vi "pickSurroundingPlatforms.vi"(9 "previousChoices":i32[][](array[numeric]), 10 "Goal \nplatform":i32, 11 "Start platform":i32) -> (3 "platform choices":i32[](array[numeric]))   [LabVIEW 2017]
panel:
  out "distance of \nchoices":dbl[](array[numeric])
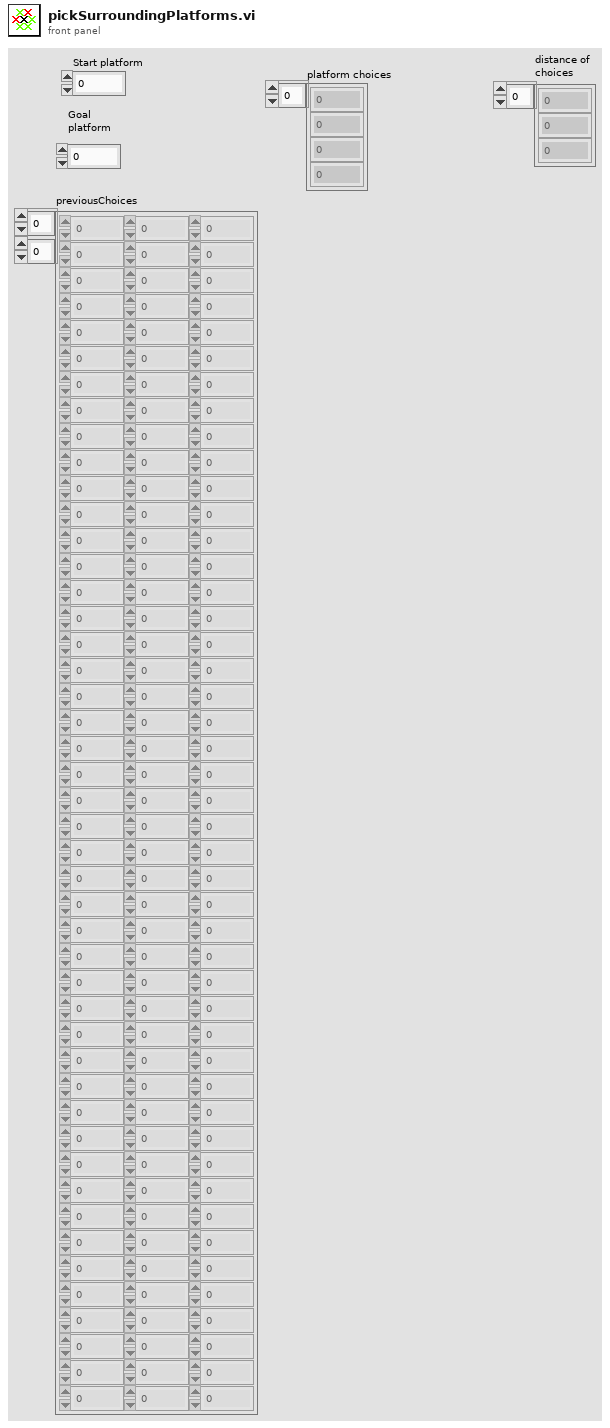
[diagram p1: front panel]
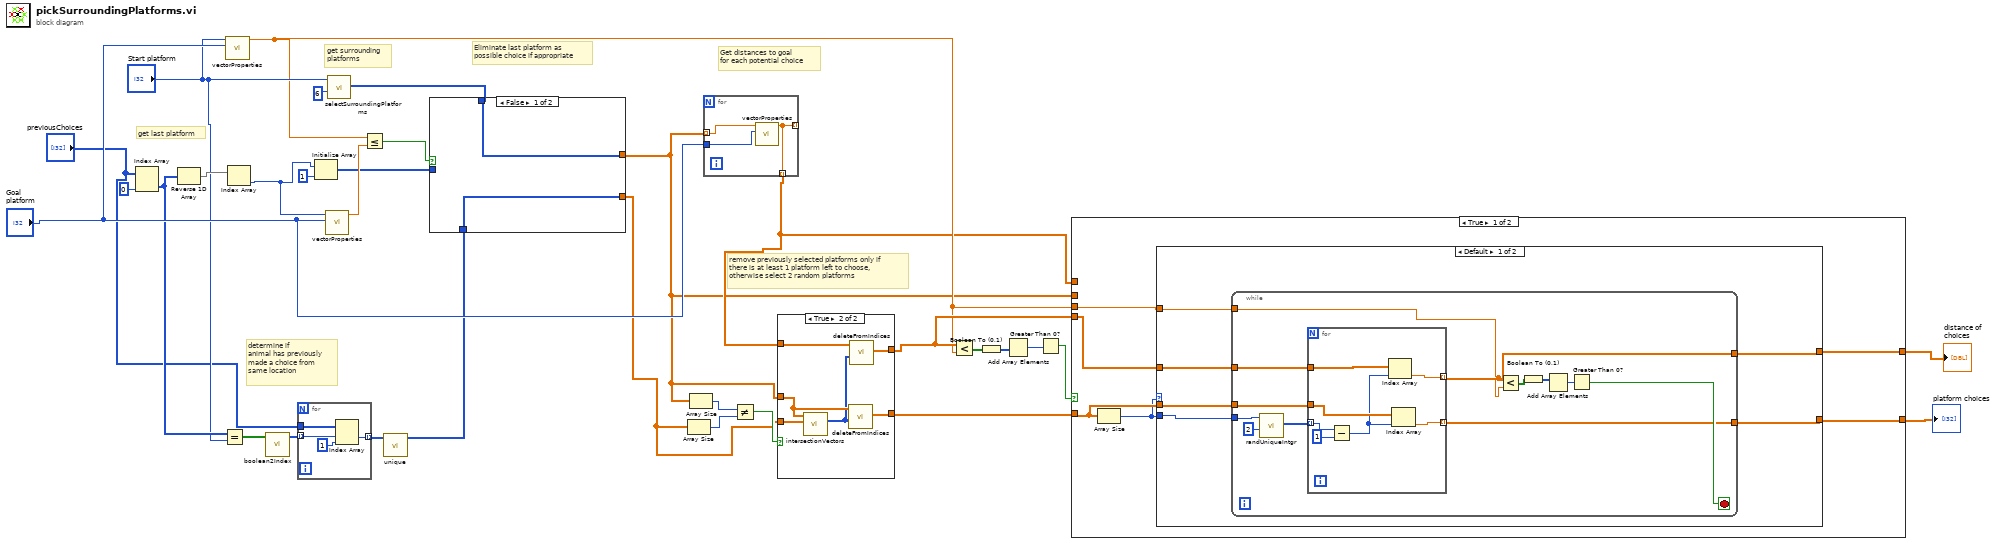
[diagram p0: block diagram]
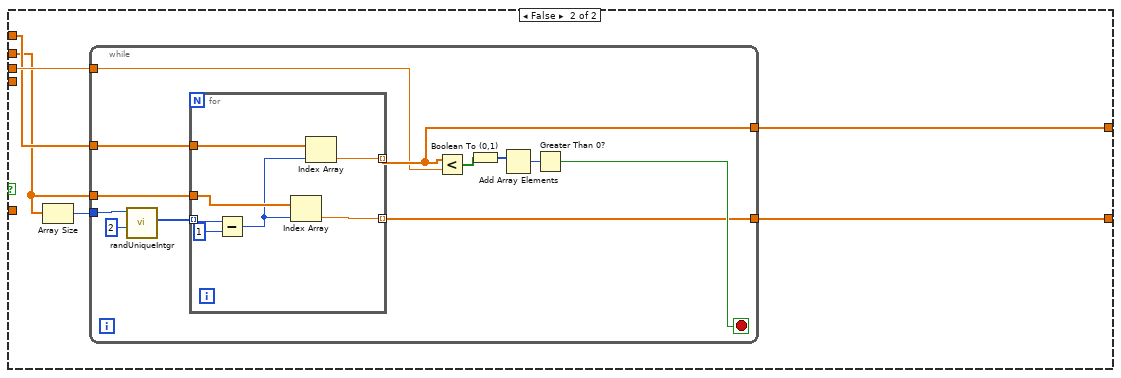
[diagram p3: hidden frame]
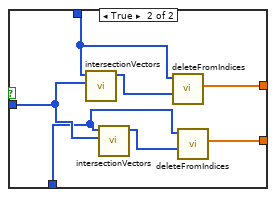
[diagram p5: hidden frame]
diagram:
  # "remove previously selected platforms only if \nthere is at least 1 platform left to choose,\notherwise select 2 random platforms"
  # "determine if \nanimal has previously \nmade a choice from \nsame location"
  # "Get distances to goal\nfor each potential choice"
  # "Eliminate last platform as \npossible choice if appropriate"
  # "get last platform"
  # "get surrounding\nplatforms"
  n1 = Index Array(array="previousChoices", index (col)=0 ("disabled index (col)")) -> (element=w20:i32[])  [unwired: 1 in]
  n2 = Reverse 1D Array(array=w20) -> (reversed array=w30:i32[])
  n3 = Equal?(x=w20, y="Start platform") -> (x = y?=w24:bool[])
  n4 = call "vectorProperties.vi"("Goal \nplatform"="Goal \nplatform", "Start \nplatform"="Start platform") -> ("vector length"=w6:dbl)  [unwired: 8 in, 1 out]
  n5 = Index Array(array=w30) -> (element=w27:i32)  [unwired: 1 in]
  n6 = call "boolean2Index.vi"("boolean"=w24) -> ("index"=w23:i32[])  [unwired: 10 in]
  n7 = for {
    tunnel: w23 -> [w35] mode=indexing
    tunnel: "previousChoices" -> [w36]
    tunnel: [w33] -> w17 mode=indexing
    n8 = Index Array(array=w36, index (row)=w35, index (col)=1) -> (element=w33:i32)
  }
  n9 = Initialize Array(w27, 1 ("dimension size")) -> (w26:i32[])
  n10 = call "vectorProperties.vi"("Goal \nplatform"="Goal \nplatform", "Start \nplatform"=w27) -> ("vector length"=w29:dbl)  [unwired: 8 in, 1 out]
  n11 = call "selectSurroundingPlatforms.vi"("Number of surrounding\nplatforms to raise"=6 ("Number of surrounding\nplatforms to raise"), "Start platform"="Start platform") -> ("Platforms \nto raise"=w16:i32[])  [unwired: 9 in]
  n12 = Less Or Equal?(x=w6, y=w29) -> (x <= y?=w28:bool)
  n13 = call "unique.vi"("Array"=w17) -> ("Array 2"=w15:i32[])  [unwired: 10 in]
  n14 = case shown="False" w28 {
    tunnel: w16 -> [w38 w44]
    tunnel: w26 -> [_ w42]
    tunnel: [w38 w43] -> w4
    tunnel: w15 -> [w37 w40]
    tunnel: [w37 w39] -> w12
    frame False {
    }
    frame True {
      n15 = call "intersectionVectors.vi"("vector2"=w42, "vector1"=w44) -> ("vector1 indices"=w45:i32[])  [unwired: 8 in, 1 out]
      n16 = call "intersectionVectors.vi"("vector2"=w42, "vector1"=w40) -> ("vector1 indices"=w41:i32[])  [unwired: 8 in, 1 out]
      n17 = call "deleteFromIndices.vi"("indices to delete"=w45, "vector"=w44) -> ("vector restricted"=w43:dbl[])  [unwired: 9 in]
      n18 = call "deleteFromIndices.vi"("indices to delete"=w41, "vector"=w40) -> ("vector restricted"=w39:dbl[])  [unwired: 9 in]
    }
  }
  n19 = Array Size(array=w12) -> (size(s)=w21:i32)
  n20 = Array Size(array=w4) -> (size(s)=w22:i32)
  n21 = for {
    tunnel: w4 -> [w48] mode=indexing
    tunnel: "Goal \nplatform" -> [w47]
    tunnel: [w46] -> _ mode=indexing
    tunnel: [w46] -> w5 mode=indexing
    n22 = call "vectorProperties.vi"("Goal \nplatform"=w47, "Start \nplatform"=w48) -> ("vector length"=w46:dbl)  [unwired: 8 in, 1 out]
  }
  n23 = Not Equal?(x=w22, y=w21) -> (x != y?=w13:bool)
  n24 = case shown="True" w13 {
    tunnel: [w50 w56] -> w14
    tunnel: w4 -> [w50 w55]
    tunnel: w12 -> [_ w54]
    tunnel: w5 -> [w49 w53]
    tunnel: [w49 w51] -> w7
    frame False {
    }
    frame True {
      n25 = call "intersectionVectors.vi"("vector2"=w54, "vector1"=w55) -> ("vector1 indices"=w52:i32[])  [unwired: 8 in, 1 out]
      n26 = call "deleteFromIndices.vi"("indices to delete"=w52, "vector"=w55) -> ("vector restricted"=w56:dbl[])  [unwired: 9 in]
      n27 = call "deleteFromIndices.vi"("indices to delete"=w52, "vector"=w53) -> ("vector restricted"=w51:dbl[])  [unwired: 9 in]
    }
  }
  n28 = Less?(x=w7, y=w6) -> (x < y?=w11:bool[])
  n29 = Boolean To (0,1)(Boolean=w11) -> (0, 1=w9:i16[])
  n30 = Add Array Elements(numeric array=w9) -> (sum=w10:i16)
  n31 = Greater Than 0?(x=w10) -> (x > 0?=w8:bool)
  n32 = case shown="True" w8 {
    tunnel: w14 -> [w62 _]
    tunnel: w7 -> [w61 _]
    tunnel: w6 -> [w60 w94]
    tunnel: [w59 w93] -> w3
    tunnel: w5 -> [_ w92]
    tunnel: w4 -> [_ w91]
    tunnel: [w58 w90] -> w2
    frame True {
      n33 = Array Size(array=w62) -> (size(s)=w57:i32)
      n34 = case shown="Default" w57 {
        tunnel: w57 -> [w68 _]
        tunnel: w62 -> [w67 w88]
        tunnel: w61 -> [w66 w89]
        tunnel: w60 -> [w65 _]
        tunnel: [w64 w88] -> w59
        tunnel: [w63 w89] -> w58
        frame Default {
          n35 = while {
            tunnel: w68 -> [w80]
            tunnel: w67 -> [w77]
            tunnel: w66 -> [w76]
            tunnel: w65 -> [w69]
            tunnel: [w71] -> w64
            tunnel: [w70] -> w63
            stop <- w72 stop-if-true
            n36 = call "randUniqueIntgr.vi"("max rand number"=w80, "Number of Outputs"=2) -> ("output"=w78:u32[])  [unwired: 8 in]
            n37 = for {
              tunnel: w78 -> [w83] mode=indexing
              tunnel: w77 -> [w87]
              tunnel: w76 -> [w86]
              tunnel: [w85] -> w70 mode=indexing
              tunnel: [w84] -> w71 mode=indexing
              n38 = Subtract(x=w83, y=u32 1) -> (x-y=w82:u32)
              n39 = Index Array(array=w86, index=w82) -> (element=w85:dbl)
              n40 = Index Array(array=w87, index=w82) -> (element=w84:dbl)
            }
            n41 = Less?(x=w70, y=w69) -> (x < y?=w73:bool[])
            n42 = Boolean To (0,1)(Boolean=w73) -> (0, 1=w75:i16[])
            n43 = Add Array Elements(numeric array=w75) -> (sum=w74:i16)
            n44 = Greater Than 0?(x=w74) -> (x > 0?=w72:bool)
          }
        }
        frame 1 {
        }
      }
    }
    frame False {
      n45 = Array Size(array=w91) -> (size(s)=w95:i32)
      n46 = while {
        tunnel: w95 -> [w107]
        tunnel: w91 -> [w104]
        tunnel: w92 -> [w103]
        tunnel: w94 -> [w96]
        tunnel: [w98] -> w93
        tunnel: [w97] -> w90
        stop <- w99 stop-if-true
        n47 = call "randUniqueIntgr.vi"("max rand number"=w107, "Number of Outputs"=2) -> ("output"=w105:u32[])  [unwired: 8 in]
        n48 = for {
          tunnel: w105 -> [w110] mode=indexing
          tunnel: w104 -> [w114]
          tunnel: w103 -> [w113]
          tunnel: [w112] -> w97 mode=indexing
          tunnel: [w111] -> w98 mode=indexing
          n49 = Subtract(x=w110, y=u32 1) -> (x-y=w109:u32)
          n50 = Index Array(array=w114, index=w109) -> (element=w111:dbl)
          n51 = Index Array(array=w113, index=w109) -> (element=w112:dbl)
        }
        n52 = Less?(x=w97, y=w96) -> (x < y?=w100:bool[])
        n53 = Boolean To (0,1)(Boolean=w100) -> (0, 1=w102:i16[])
        n54 = Add Array Elements(numeric array=w102) -> (sum=w101:i16)
        n55 = Greater Than 0?(x=w101) -> (x > 0?=w99:bool)
      }
    }
  }
  "platform choices" <- w3
  "distance of \nchoices" <- w2
